vi "errorQuery.vi"(8 "error in (no error)":errorcluster, 10 "VISA resource name":refnum<visa-resource-name>, 11 "Electrometer in":refnum<class "Electrometer.lvclass">) -> (0 "error out":errorcluster, 1 "Error Message":string, 2 "Error Code":i32[](array[numeric]), 3 "Electrometer out":refnum<class "Electrometer.lvclass">)   [LabVIEW 2016, in "Electrometer.lvclass"]
uses:
  Electrometer.lvclass
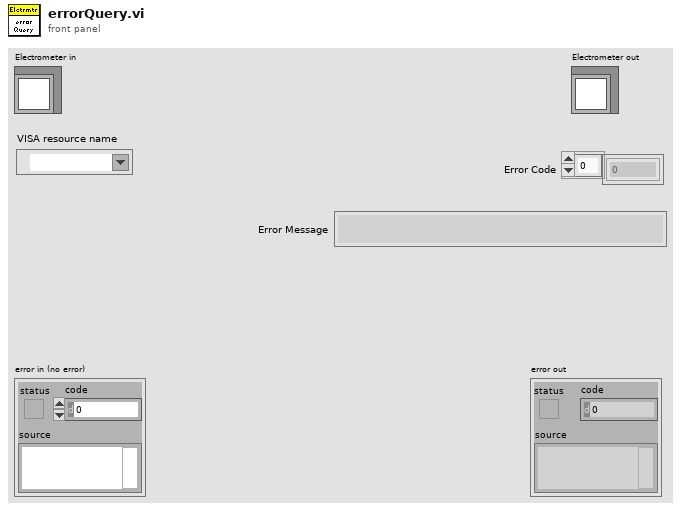
[diagram p1: front panel]
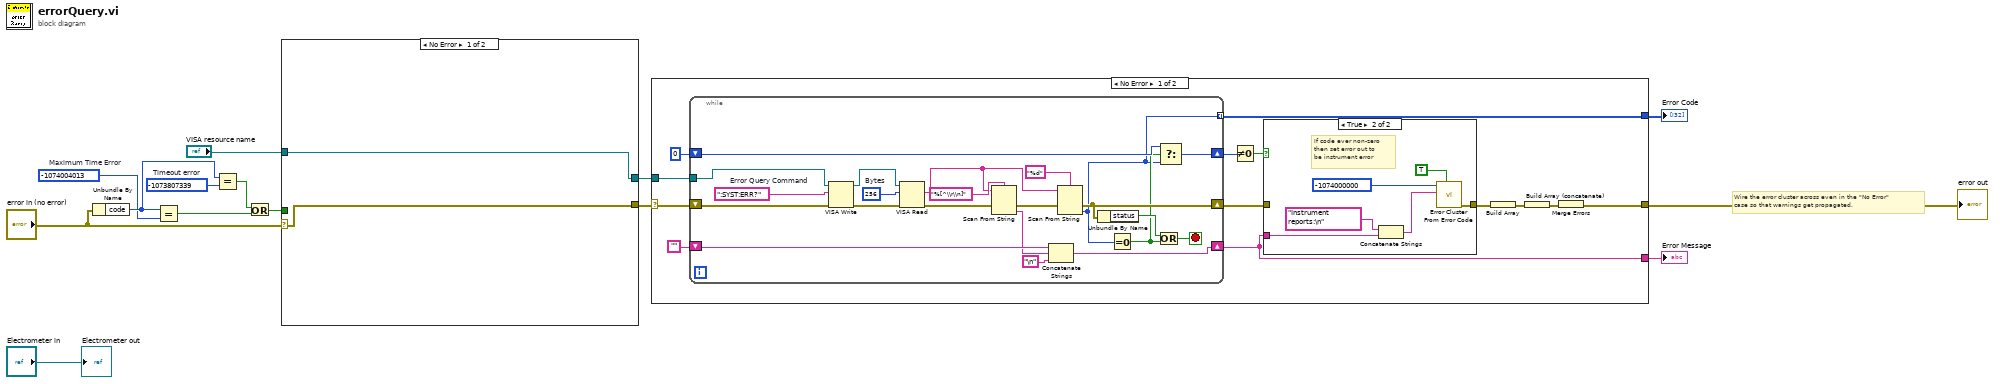
[diagram p0: block diagram]
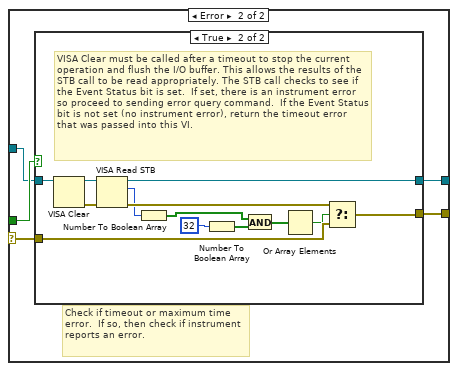
[diagram p2: hidden frame]
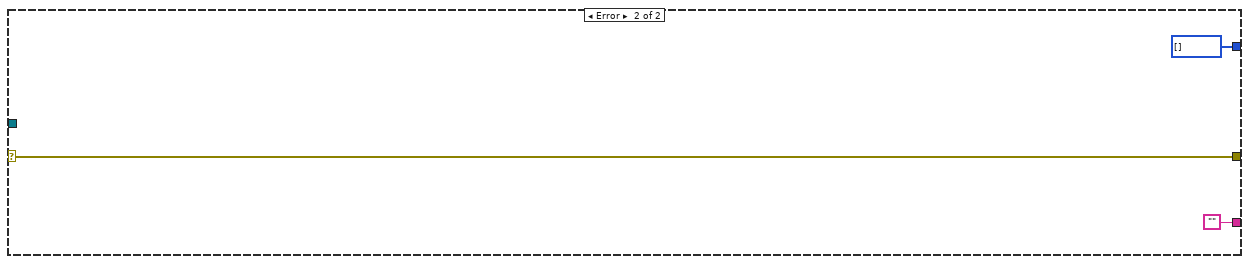
[diagram p5: hidden frame]
diagram:
  w9 = -1074004013  # Maximum Time Error
  w11 = -1073807339  # Timeout error
  # "Wire the error cluster across even in the \"No Error\"\ncase so that warnings get propagated."
  n1 = Unbundle By Name("error in (no error)") -> ("code"=w10:i32)
  n2 = Equal?(x=w10, y=w9) -> (x = y?=w8:bool)
  n3 = Equal?(x=w10, y=w11) -> (x = y?=w7:bool)
  n4 = Or(x=w7, y=w8) -> (x .or. y?=w6:bool)
  n5 = case shown="No Error" "error in (no error)" {
    selector: "error in (no error)" -> [w16 w20]
    tunnel: [w15 w21] -> w12
    tunnel: [w16 w19] -> w13
    tunnel: w6 -> [_ w18]
    tunnel: "VISA resource name" -> [w15 w17]
    frame No Error {
    }
    frame Error {
      # "Check if timeout or maximum time error.  If so, then check if instrument reports an error."
      n6 = case shown="True" w18 {
        tunnel: [w22 w27] -> w21
        tunnel: w20 -> [w23 w32]
        tunnel: [w23 w31] -> w19
        tunnel: w17 -> [w22 w24]
        frame False {
          # "Error code not a timeout, so best to pass on to user."
        }
        frame True {
          # "VISA Clear must be called after a timeout to stop the current operation and flush the I/O buffer. This allows the results of the  STB call to be read appropriately. The STB call checks to see if the Event Status bit is set.  If set, there is an instrument error so proceed to sending error query command.  If the Event Status bit is not set (no instrument error), return the timeout error that was passed into this VI."
          n7 = VISA Clear(VISA resource name=w24) -> (VISA resource name out=w29:refnum<visa-resource-name>, error out=w28:errorcluster)  [unwired: 1 in]
          n8 = VISA Read STB(8:w28, 11:w29) -> (0:w26:errorcluster, 2:w25:u16, 3:w27:refnum<visa-resource-name>)
          n9 = Number To Boolean Array(number=w25) -> (Boolean array=w33:bool[])
          n10 = Number To Boolean Array(number=32) -> (Boolean array=w35:bool[])
          n11 = And(x=w33, y=w35) -> (x .and. y?=w34:bool[])
          n12 = Or Array Elements(Boolean array=w34) -> (logical OR=w30:bool)
          n13 = Select(t=w26, s=w30, f=w32) -> (s? t:f=w31:errorcluster)
        }
      }
    }
  }
  n14 = case shown="No Error" w13 {
    selector: w13 -> [w39 w79]
    tunnel: w12 -> [w49 _]
    tunnel: [w47 w79] -> w3
    tunnel: [w42 ""] -> w2
    tunnel: [w41 i32[] []] -> w1
    frame No Error {
      n15 = while {
        tunnel: w49 -> [w78]
        shift-right: [w67] -> w42
        shift-left: "" -> [w70]
        shift-right: [w65] -> w43
        shift-left: 0 -> [w66]
        shift-right: [w63] -> w40
        shift-left: w39 -> [w64]
        tunnel: [w58] -> w41 mode=indexing
        stop <- w73 stop-if-true
        w76 = u32 256  # Bytes
        w75 = ":SYST:ERR?"  # Error Query Command
        n16 = VISA Write(VISA resource name=w78, write buffer=w75, error in (no error)=w64) -> (VISA resource name out=w77:refnum<visa-resource-name>, error out=w57:errorcluster)  [unwired: 1 out]
        n17 = VISA Read(VISA resource name=w77, byte count=w76, error in (no error)=w57) -> (read buffer=w71:string, error out=w62:errorcluster)  [unwired: 2 out]
        n18 = Scan From String(format string="%[^\\r\\n]", input string=w71, error in=w62) -> (error out=w61:errorcluster, output 1=w68:string)  [unwired: 2 in, 2 out]
        n19 = Concatenate Strings(w70, w68, "\n") -> (w67:string)
        n20 = Scan From String(format string="%d", input string=w71, error in=w61) -> (error out=w63:errorcluster, output 1=w58:i32)  [unwired: 2 in, 2 out]
        n21 = Unbundle By Name(w63) -> ("status"=w60:bool)
        n22 = Equal To 0?(x=w58) -> (x = 0?=w59:bool)
        n23 = Or(x=w60, y=w59) -> (x .or. y?=w73:bool)
        n24 = Select(t=w66, s=w59, f=w58) -> (s? t:f=w65:i32)
      }
      n25 = Not Equal To 0?(x=w43) -> (x != 0?=w45:bool)
      n26 = case shown="True" w45 {
        tunnel: w42 -> [_ w55]
        tunnel: [w50 w51] -> w44
        tunnel: w40 -> [w50 _]
        frame False {
        }
        frame True {
          # "If code ever non-zero\nthen set error out to\nbe instrument error"
          n27 = Concatenate Strings("Instrument reports:\n" ("Source"), w55) -> (w52:string)
          n28 = call <vilib>:"Error Cluster From Error Code.vi"("show call chain? (False)"=TRUE, "error message (\"\")"=w52, "error code (0)"=-1074000000 ("Code")) -> ("error out"=w51:errorcluster)  [unwired: 6 in]
        }
      }
      n29 = Build Array(w44) -> (w38:errorcluster[])
      n30 = Build Array (concatenate)(w38) -> (w37:errorcluster[])
      n31 = Merge Errors(w37) -> (w47:errorcluster)
    }
    frame Error {
    }
  }
  "error out" <- w3
  "Error Message" <- w2
  "Error Code" <- w1
  "Electrometer out" <- "Electrometer in"
